vi "Link_File Names.vi"() -> (0 "Unlink file name":string, 1 "Link file name":string)   [LabVIEW 2019, in "AutoMenuCreator.lvlib"]
uses:
  AutoMenuCreator.lvlib
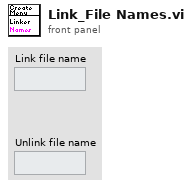
[diagram p1: front panel]
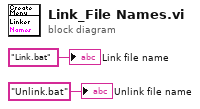
[diagram p0: block diagram]
diagram:
  "Unlink file name" <- "Unlink.bat" ("string")
  "Link file name" <- "Link.bat" ("string")
